vi "Test program 2.vi"() -> ()   [LabVIEW 2013, in "Keithly user program.lvlib"]
doc: "Example VI showing how to source a DC current."
uses:
  Keithly user program.lvlib
  Typedefs/KE622x -- On Off Control.ctl
  Configure/Output/Typedefs/KE6221 -- Output Response.ctl
  Configure/Source/Typedefs/KE622x -- Current Range.ctl
  Configure/Source/Typedefs/KE622x -- Current Level.ctl
  Configure/Source/Typedefs/KE622x -- Voltage Limit.ctl
  Configure/Utility/Typedefs/KE622x -- Instrument Type.ctl
panel:
  in  "Instrument Type":T1=enum."KE6221"
  in  "Output State":T2
  in  "Voltage Limit (V)":T3=10.0 min=0.1 max=105.0 step=0.01 format="%.2p"
  in  "Current Level (A)":T4=0.001 min=-0.105 max=0.105 format="%.4p"
  in  "Current Range":T5={"Auto Range?"=FALSE, "Man / Selected\n        Range"=enum."2mA"}
  in  "Output Response":T6=enum."Slow"
  in  "Analog Filter State":T2
  in  "Turn Off Output If Voltage Limit?":bool=TRUE
  out "error out":errorcluster
  out "Voltage Limit?":bool
  out "Interlock Tripped?":bool
  in  "Check For SCPI Errors? (T)":bool=TRUE
  in  "VISA resource name":refnum<visa-resource-name>
  # "*** NOTE:  only apples to KE6221"
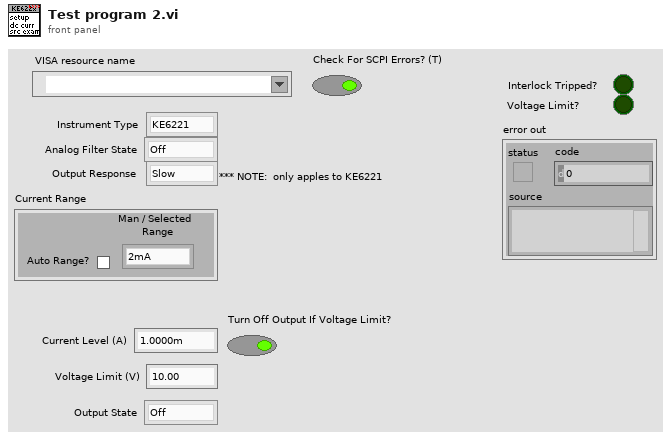
[diagram p1: front panel]
types:
  T1 = typedef "Keithly user program.lvlib/KE622x -- Instrument Type.ctl" = enum16{"KE6220", "KE6221"}
  T2 = typedef "Keithly user program.lvlib/KE622x -- On Off Control.ctl" = enum16{"Off", "On"}
  T3 = typedef "Keithly user program.lvlib/KE622x -- Voltage Limit.ctl" = dbl
  T4 = typedef "Keithly user program.lvlib/KE622x -- Current Level.ctl" = dbl
  T5 = typedef "Keithly user program.lvlib/KE622x -- Current Range.ctl" = cluster{"Auto Range?":bool, "Man / Selected\n        Range":enum16{"2nA", "20nA", "200nA", "2uA", "20uA", "200uA", "2mA", "20mA", "100mA"}}
  T6 = typedef "Keithly user program.lvlib/KE6221 -- Output Response.ctl" = enum16{"Fast", "Slow"}
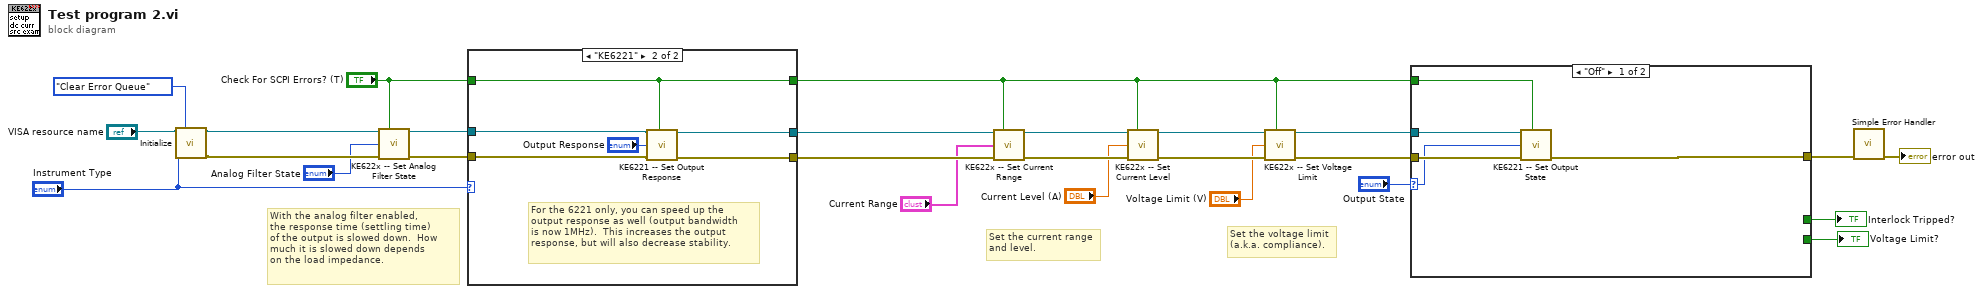
[diagram p0: block diagram]
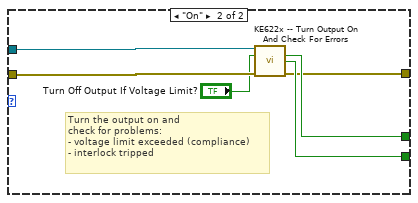
[diagram p2: hidden frame]
diagram:
  # "Set the voltage limit\n(a.k.a. compliance)."
  # "Set the current range\nand level."
  # "With the analog filter enabled,\nthe response time (settling time)\nof the output is slowed down.  How\nmuch it is slowed down depends\non the load impedance."
  n1 = call "Initialize.vi"("VISA resource name"="VISA resource name", "Error Queue Option"=enum16{"Clear Error Queue", "Error Query"}."Clear Error Queue", "Instrument Type"="Instrument Type") -> ("VISA resource name out"=w20:refnum<visa-resource-name>, "error out"=w17:errorcluster)  [unwired: 11 in]
  n2 = call "KE622x -- Set Analog Filter State.vi"("Resource In"=w20, "Check For SCPI Errors? (T)"="Check For SCPI Errors? (T)", "Analog Filter State"="Analog Filter State", "error in (no error)"=w17) -> ("Resource Out (dupl)"=w19:refnum<visa-resource-name>, "error out"=w16:errorcluster)  [unwired: 10 in]
  n3 = case shown="\"KE6221\"" "Instrument Type" {
    tunnel: w19 -> [w28 w34]
    tunnel: w16 -> [w27 w33]
    tunnel: [w28 w35] -> w14
    tunnel: "Check For SCPI Errors? (T)" -> [w29 w31]
    tunnel: [w29 w31] -> w6
    tunnel: [w27 w32] -> w13
    frame "KE6220" {
    }
    frame "KE6221" {
      # "For the 6221 only, you can speed up the\noutput response as well (output bandwidth\nis now 1MHz).  This increases the output\nresponse, but will also decrease stability."
      n4 = call "KE6221 -- Set Output Response.vi"("Resource In"=w34, "Check For SCPI Errors? (T)"=w31, "KE6221 Output Response"="Output Response", "error in (no error)"=w33) -> ("Resource Out (dupl)"=w35:refnum<visa-resource-name>, "error out"=w32:errorcluster)  [unwired: 10 in]
    }
  }
  n5 = call "KE622x -- Set Current Range.vi"("Resource In"=w14, "Check For SCPI Errors? (T)"=w6, "Current Range"="Current Range", "error in (no error)"=w13) -> ("Resource Out (dupl)"=w11:refnum<visa-resource-name>, "error out"=w10:errorcluster)  [unwired: 10 in]
  n6 = call "KE622x -- Set Current Level.vi"("Resource In"=w11, "Check For SCPI Errors? (T)"=w6, "Current Level (A)"="Current Level (A)", "error in (no error)"=w10) -> ("Resource Out (dupl)"=w8:refnum<visa-resource-name>, "error out"=w5:errorcluster)  [unwired: 10 in]
  n7 = call "KE622x -- Set Voltage Limit.vi"("Resource In"=w8, "Check For SCPI Errors? (T)"=w6, "Voltage Limit (V)"="Voltage Limit (V)", "error in (no error)"=w5) -> ("Resource Out (dupl)"=w7:refnum<visa-resource-name>, "error out"=w4:errorcluster)  [unwired: 10 in]
  n8 = case shown="\"Off\"" "Output State" {
    selector: "Output State" -> [w36 _]
    tunnel: w7 -> [w39 w46]
    tunnel: w4 -> [w38 w45]
    tunnel: [w37 w41] -> w26
    tunnel: w6 -> [w40 _]
    tunnel: [_ w43] -> w24
    tunnel: [_ w42] -> w23
    frame "Off" {
      n9 = call "KE6221 -- Set Output State.vi"("Resource In"=w39, "Check For SCPI Errors? (T)"=w40, "Output State"=w36, "error in (no error)"=w38) -> ("error out"=w37:errorcluster)  [unwired: 10 in, 1 out]
    }
    frame "On" {
      # "Turn the output on and\ncheck for problems:\n- voltage limit exceeded (compliance)\n- interlock tripped"
      n10 = call "KE622x -- Turn Output On And Check For Errors.vi"("Resource In"=w46, "Turn Off Output If Compliance?"="Turn Off Output If Voltage Limit?", "error in (no error)"=w45) -> ("Interlock Tripped?"=w43:bool, "Compliance?"=w42:bool, "error out"=w41:errorcluster)  [unwired: 9 in, 1 out]
    }
  }
  "Interlock Tripped?" <- w24
  "Voltage Limit?" <- w23
  n11 = call <vilib>:"Simple Error Handler.vi"("error in (no error)"=w26) -> ("error out"=→"error out":errorcluster)  [unwired: 4 in, 4 out]
